vi "Main_TwoLoops.vi"() -> ()   [LabVIEW 2018]
uses:
  SubVIs/ENUMs/StateENUM.ctl
  <vilib>/Instr/_visa.llb/VISA Configure Serial Port (Instr).vi
  <vilib>/ptbypt/NI_PtbyPt.lvlib
panel:
  out "Waveform Chart":dbl(graph)
  in  "Check Center":bool
  out "Step":i32
  in  "Increase Step":bool
  in  "Decrease Step":bool
  out "Center":i32
  out "LoopCount":i32
  in  "Jitter Up":bool
  in  "Jitter Down":bool
  out "Command Buffer":string
  in  "stop":bool
  out "Current Time":timestamp format="%<%I:%M:%S %p | %m/%d/%y>T"
  in  "VISA resource name":refnum<visa-resource-name>="COM9"
  in  "Up Button":bool
  in  "Down Button":bool
  # "Manual\nAdjustment"
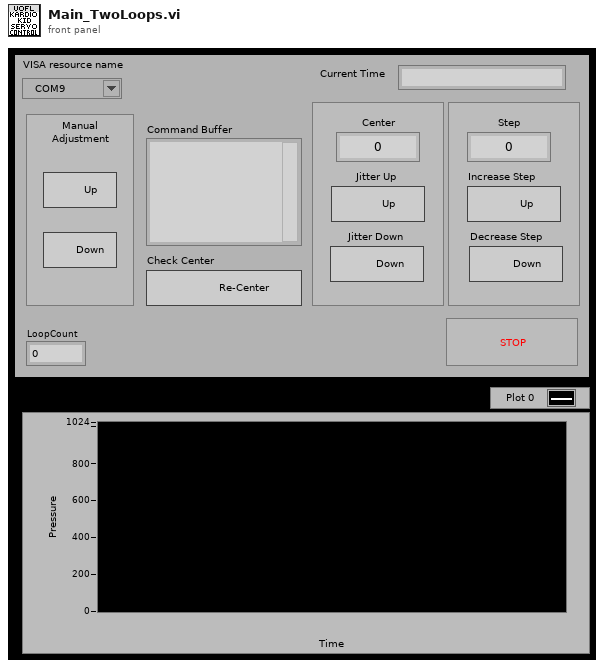
[diagram p1: front panel]
types:
  T1 = typedef "StateENUM.ctl" = enum16{"Init", "Idle", "MoveUp", "MoveDown", "JitterUp", "JitterDown", "IncreaseStep", "DecreaseStep", "CheckCenter", "ReadSerial", "ScanData", "Shutdown"}
  T2 = cluster{"State":T1, "Stop":bool, "error out":errorcluster}
  T3 = typedef "MoveCommands.ctl" = cluster{"MoveUp":string, "MoveDown":string, "JitterUp":string, "JitterDown":string, "IncStep":string, "DecStep":string, "ChkCenter":string}
  T4 = cluster{"VISA resource name out":refnum<visa-resource-name>, "error out":errorcluster, "State":T1, "Stop":bool, "Buffer":string, "Center":i32, "Step":i32, "SerialIncoming?":bool, "MoveCommands":T3}
  T5 = cluster{"Command Buffer":refnum<vi>, "Jitter Up":refnum<vi>, "Jitter Down":refnum<vi>, "Increase Step":refnum<vi>, "Decrease Step":refnum<vi>}
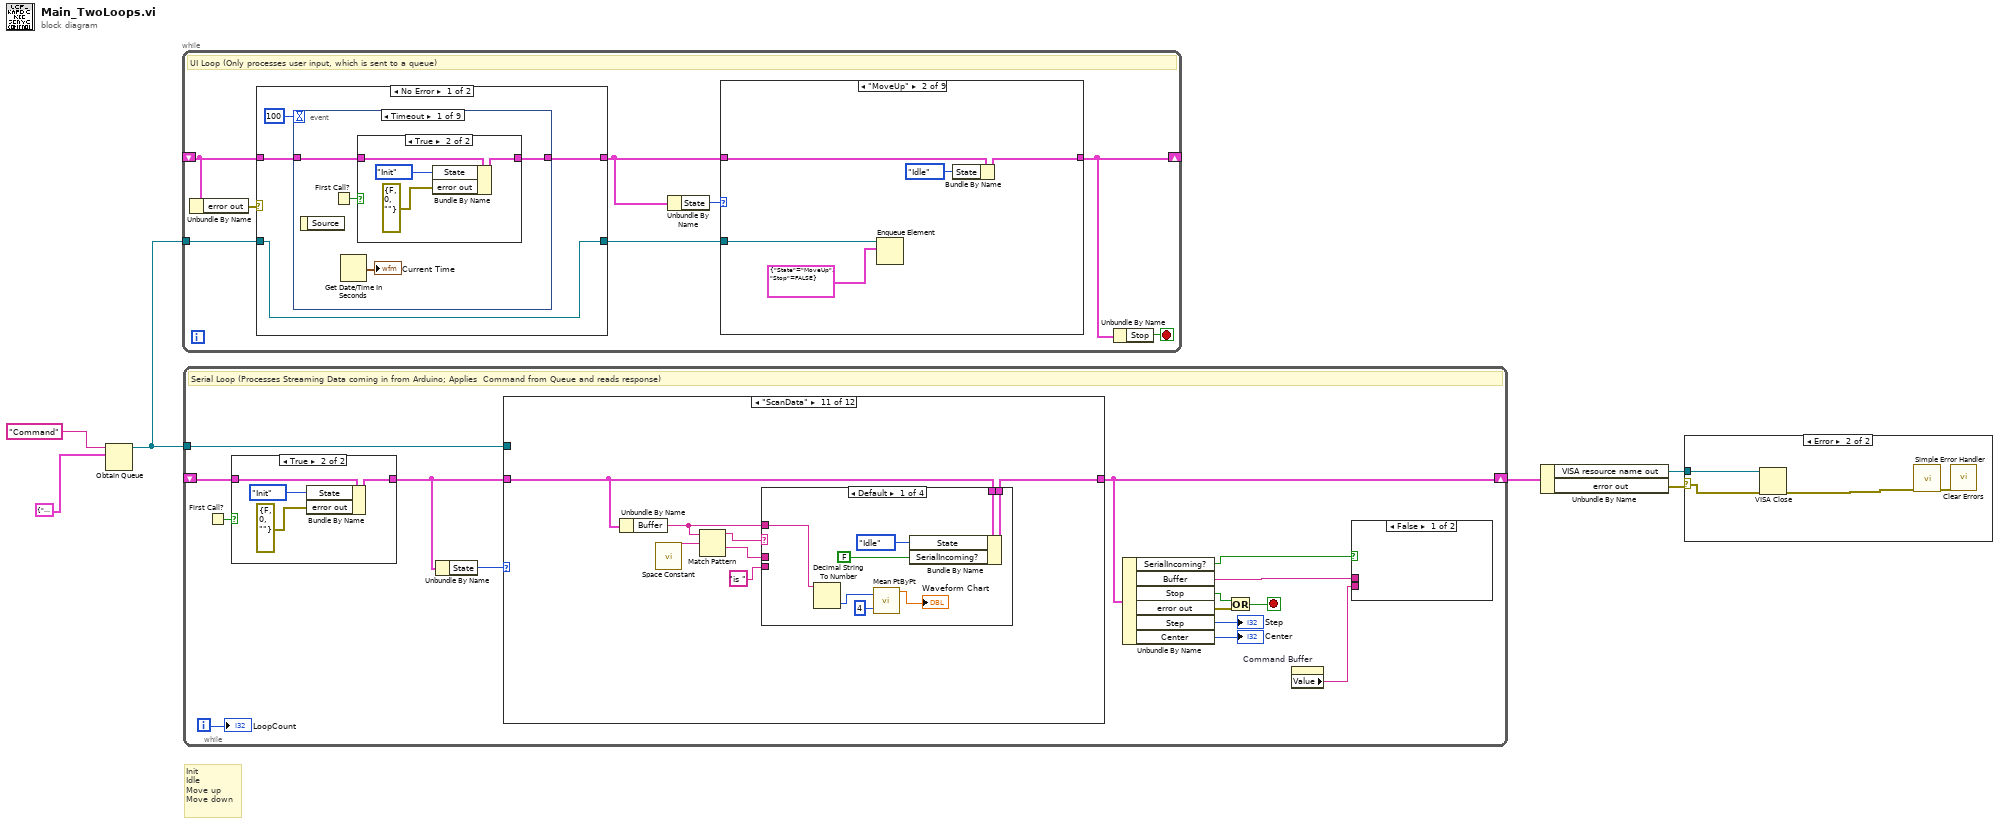
[diagram p0: block diagram]
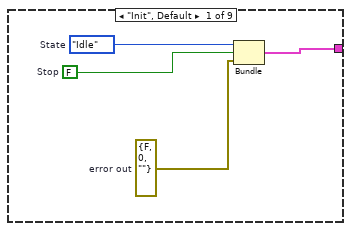
[diagram p2: hidden frame]
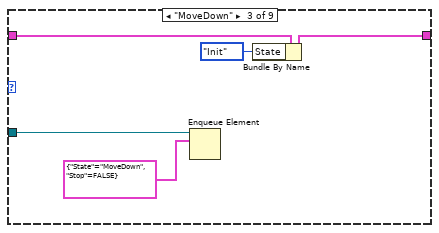
[diagram p3: hidden frame]
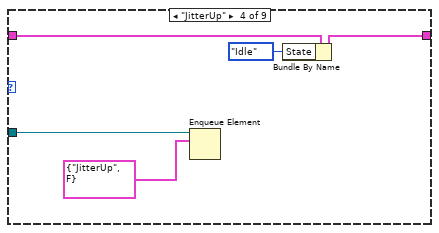
[diagram p4: hidden frame]
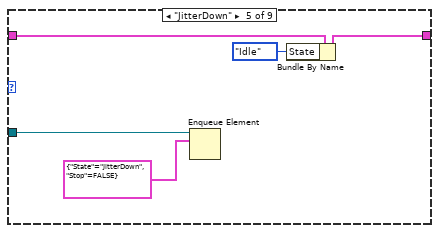
[diagram p5: hidden frame]
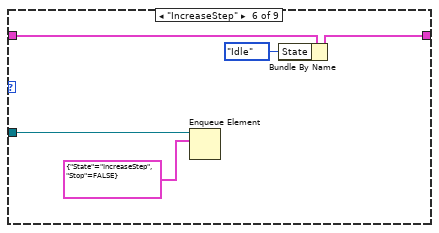
[diagram p6: hidden frame]
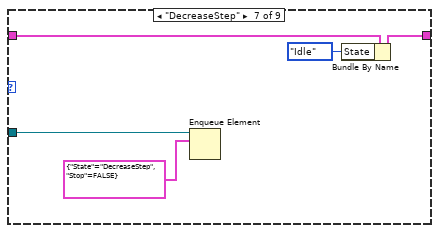
[diagram p7: hidden frame]
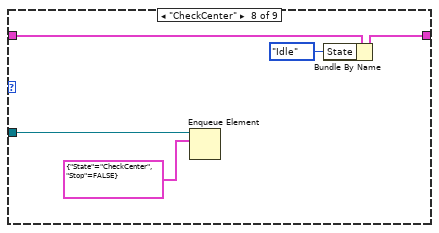
[diagram p8: hidden frame]
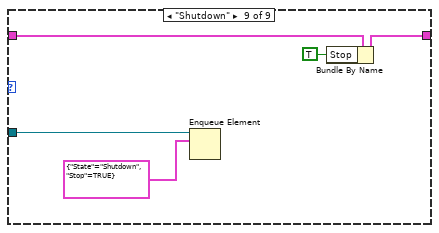
[diagram p9: hidden frame]
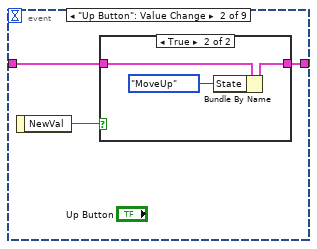
[diagram p11: hidden frame]
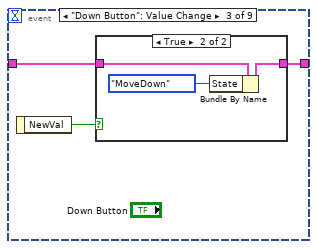
[diagram p13: hidden frame]
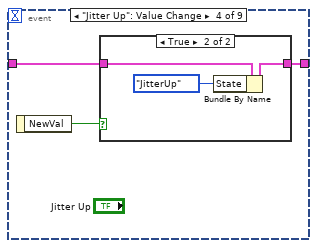
[diagram p15: hidden frame]
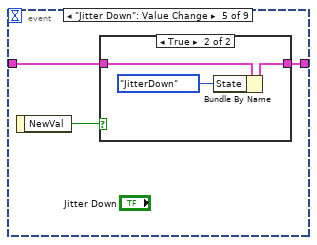
[diagram p17: hidden frame]
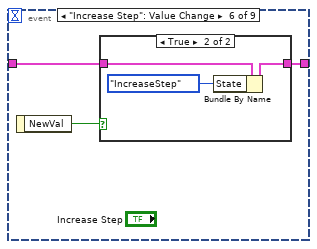
[diagram p19: hidden frame]
diagram:
  # "Init\nIdle\nMove up\nMove down"
  n1 = Obtain Queue(name (unnamed)="Command", element data type=cluster{"State":T1, "Stop":bool} {"State"=enum."ReadSerial", "Stop"=FALSE}) -> (queue out=w1:refnum<queue>)  [unwired: 3 in, 2 out]
  n2 = while {
    shift-right: [w13] -> _
    shift-left: _ -> [w10]
    tunnel: w1 -> [w8]
    stop <- w12 stop-if-true
    # "UI Loop (Only processes user input, which is sent to a queue)"
    n3 = Unbundle By Name(w10) -> ("error out"=w9:errorcluster)
    n4 = case shown="No Error" w9 {
      tunnel: w10 -> [w60 w134]
      tunnel: [w61 w130] -> w14
      tunnel: w8 -> [w59 w128]
      tunnel: [w59 w128] -> w7
      frame No Error {
        n5 = event shown="[0] Timeout" {
          selector: _ -> [_ _ _ _ _ _ _ _ _]
          dyn-events: _ -> [_ _ _ _ _ _ _ _ _]
          timeout: 100 -> [_ _ _ _ _ _ _ _ _]
          tunnel: w60 -> [w64 w74 w80 w88 w95 w102 w109 w116 w122]
          tunnel: [w63 w72 w79 w86 w93 w100 w107 w114 w121] -> w61
          event Timeout {
            n6 = event-data() -> ()  [unwired: 1 in, 1 out]
            n7 = First Call?() -> (First Call?: T/F=w65:bool)
            n8 = Get Date/Time In Seconds() -> (seconds since 1Jan1904=→"Current Time":timestamp)
            n9 = case shown="True" w65 {
              tunnel: [w67 w70] -> w63
              tunnel: w64 -> [w67 w71]
              frame False {
              }
              frame True {
                n10 = Bundle By Name(cluster=w71, "State"=StateENUM."Init", "error out"=errorcluster {"status"=FALSE, "code"=0, "source"=""}) -> (w70:T2)
              }
            }
          }
          event "Up Button": Value Change {
            n11 = event-data() -> ("NewVal"=w73:bool)  [unwired: 1 in]
            n12 = case shown="True" w73 {
              tunnel: w74 -> [w75 w78]
              tunnel: [w75 w77] -> w72
              frame False {
              }
              frame True {
                n13 = Bundle By Name(cluster=w78, "State"=StateENUM."MoveUp") -> (w77:T2)
              }
            }
          }
          event "Down Button": Value Change {
            n14 = event-data() -> ("NewVal"=w81:bool)  [unwired: 1 in]
            n15 = case shown="True" w81 {
              tunnel: w80 -> [w82 w85]
              tunnel: [w82 w84] -> w79
              frame False {
              }
              frame True {
                n16 = Bundle By Name(cluster=w85, "State"=StateENUM."MoveDown") -> (w84:T2)
              }
            }
          }
          event "Jitter Up": Value Change {
            n17 = event-data() -> ("NewVal"=w87:bool)  [unwired: 1 in]
            n18 = case shown="True" w87 {
              tunnel: w88 -> [w89 w92]
              tunnel: [w89 w91] -> w86
              frame False {
              }
              frame True {
                n19 = Bundle By Name(cluster=w92, "State"=StateENUM."JitterUp") -> (w91:T2)
              }
            }
          }
          event "Jitter Down": Value Change {
            n20 = event-data() -> ("NewVal"=w94:bool)  [unwired: 1 in]
            n21 = case shown="True" w94 {
              tunnel: w95 -> [w96 w99]
              tunnel: [w96 w98] -> w93
              frame False {
              }
              frame True {
                n22 = Bundle By Name(cluster=w99, "State"=StateENUM."JitterDown") -> (w98:T2)
              }
            }
          }
          event "Increase Step": Value Change {
            n23 = event-data() -> ("NewVal"=w101:bool)  [unwired: 1 in]
            n24 = case shown="True" w101 {
              tunnel: w102 -> [w103 w106]
              tunnel: [w103 w105] -> w100
              frame False {
              }
              frame True {
                n25 = Bundle By Name(cluster=w106, "State"=StateENUM."IncreaseStep") -> (w105:T2)
              }
            }
          }
          event "Decrease Step": Value Change {
            n26 = event-data() -> ("NewVal"=w108:bool)  [unwired: 1 in]
            n27 = case shown="True" w108 {
              tunnel: w109 -> [w110 w113]
              tunnel: [w110 w112] -> w107
              frame False {
              }
              frame True {
                n28 = Bundle By Name(cluster=w113, "State"=StateENUM."DecreaseStep") -> (w112:T2)
              }
            }
          }
          event "Check Center": Value Change {
            n29 = event-data() -> ("NewVal"=w115:bool)  [unwired: 1 in]
            n30 = case shown="True" w115 {
              tunnel: w116 -> [w117 w120]
              tunnel: [w117 w119] -> w114
              frame False {
              }
              frame True {
                n31 = Bundle By Name(cluster=w120, "State"=StateENUM."CheckCenter") -> (w119:T2)
              }
            }
          }
          event "stop": Value Change {
            n32 = event-data() -> ("NewVal"=w123:bool)  [unwired: 1 in]
            n33 = case shown="True" w123 {
              tunnel: w122 -> [w124 w127]
              tunnel: [w124 w126] -> w121
              frame False {
              }
              frame True {
                n34 = Bundle By Name(cluster=w127, "State"=StateENUM."Shutdown") -> (w126:T2)
              }
            }
          }
        }
      }
      frame Error {
        n35 = Unbundle By Name(w134) -> ("error out"=w133:errorcluster)
        n36 = call <vilib>:"Simple Error Handler.vi"("error in (no error)"=w133) -> ("code out"=w131:i32, "error out"=w132:errorcluster)  [unwired: 4 in, 3 out]
        n37 = call <vilib>:"Clear Errors.vi"("error in (no error)"=w132, "specific error code to clear (0: all)"=w131) -> ()  [unwired: 4 in, 2 out]
        n38 = Bundle By Name(cluster=w134, "State"=StateENUM."Shutdown") -> (w130:T2)
      }
    }
    n39 = Unbundle By Name(w14) -> ("State"=w11:T1)
    n40 = case shown="\"MoveUp\"" w11 {
      tunnel: w14 -> [_ w21 w26 w31 w36 w41 w46 w51 w56]
      tunnel: [w16 w20 w25 w30 w35 w40 w45 w50 w55] -> w13
      tunnel: w7 -> [_ w23 w28 w33 w38 w43 w48 w53 w58]
      frame "Init", Default {
        w15 = errorcluster {"status"=FALSE, "code"=0, "source"=""}  # error out
        w17 = FALSE  # Stop
        w18 = StateENUM."Idle"  # State
        n41 = Bundle("State"=w18, "Stop"=w17, "error out"=w15) -> (w16:T2)  [unwired: 1 in]
      }
      frame "MoveUp" {
        n42 = Enqueue Element(queue=w23, element=cluster{"State":T1, "Stop":bool} {"State"=enum."MoveUp", "Stop"=FALSE}) -> ()  [unwired: 2 in, 3 out]
        n43 = Bundle By Name(cluster=w21, "State"=StateENUM."Idle") -> (w20:T2)
      }
      frame "MoveDown" {
        n44 = Enqueue Element(queue=w28, element=cluster{"State":T1, "Stop":bool} {"State"=enum."MoveDown", "Stop"=FALSE}) -> ()  [unwired: 2 in, 3 out]
        n45 = Bundle By Name(cluster=w26, "State"=StateENUM."Init") -> (w25:T2)
      }
      frame "JitterUp" {
        n46 = Enqueue Element(queue=w33, element=cluster{"State":T1, "Stop":bool} {"State"=enum."JitterUp", "Stop"=FALSE}) -> ()  [unwired: 2 in, 3 out]
        n47 = Bundle By Name(cluster=w31, "State"=StateENUM."Idle") -> (w30:T2)
      }
      frame "JitterDown" {
        n48 = Enqueue Element(queue=w38, element=cluster{"State":T1, "Stop":bool} {"State"=enum."JitterDown", "Stop"=FALSE}) -> ()  [unwired: 2 in, 3 out]
        n49 = Bundle By Name(cluster=w36, "State"=StateENUM."Idle") -> (w35:T2)
      }
      frame "IncreaseStep" {
        n50 = Enqueue Element(queue=w43, element=cluster{"State":T1, "Stop":bool} {"State"=enum."IncreaseStep", "Stop"=FALSE}) -> ()  [unwired: 2 in, 3 out]
        n51 = Bundle By Name(cluster=w41, "State"=StateENUM."Idle") -> (w40:T2)
      }
      frame "DecreaseStep" {
        n52 = Enqueue Element(queue=w48, element=cluster{"State":T1, "Stop":bool} {"State"=enum."DecreaseStep", "Stop"=FALSE}) -> ()  [unwired: 2 in, 3 out]
        n53 = Bundle By Name(cluster=w46, "State"=StateENUM."Idle") -> (w45:T2)
      }
      frame "CheckCenter" {
        n54 = Enqueue Element(queue=w53, element=cluster{"State":T1, "Stop":bool} {"State"=enum."CheckCenter", "Stop"=FALSE}) -> ()  [unwired: 2 in, 3 out]
        n55 = Bundle By Name(cluster=w51, "State"=StateENUM."Idle") -> (w50:T2)
      }
      frame "Shutdown" {
        n56 = Enqueue Element(queue=w58, element=cluster{"State":T1, "Stop":bool} {"State"=enum."Shutdown", "Stop"=TRUE}) -> ()  [unwired: 2 in, 3 out]
        n57 = Bundle By Name(cluster=w56, "Stop"=TRUE) -> (w55:T2)
      }
    }
    n58 = Unbundle By Name(w13) -> ("Stop"=w12:bool)
  }
  n59 = while {
    shift-right: [w148] -> w6
    shift-left: _ -> [w137]
    tunnel: w1 -> [w135]
    i -> [w147]
    stop <- w146 stop-if-true
    # "Serial Loop (Processes Streaming Data coming in from Arduino; Applies  Command from Queue and reads response)"
    n60 = First Call?() -> (First Call?: T/F=w138:bool)
    n61 = case shown="True" w138 {
      tunnel: [w150 w153] -> w136
      tunnel: w137 -> [w150 w154]
      frame False {
      }
      frame True {
        n62 = Bundle By Name(cluster=w154, "State"=StateENUM."Init", "error out"=errorcluster {"status"=FALSE, "code"=0, "source"=""}) -> (w153:T4)
      }
    }
    n63 = Unbundle By Name(w136) -> ("State"=w149:T1)
    n64 = case shown="\"ScanData\"" w149 {
      tunnel: [w178 w183 w206 w213 w221 w230 w237 w244 w251 w266 w284 w323] -> w148
      tunnel: w136 -> [_ w184 w207 w214 w223 w232 w239 w246 w253 w267 w285 w325]
      tunnel: w135 -> [_ w182 _ _ _ _ _ _ _ _ _ w318]
      frame "Init", Default {
        w166 = FALSE  # SerialIncoming?
        w168 = 50  # Step
        w169 = 1500  # Center
        w171 = ""  # Buffer
        w176 = FALSE  # Stop
        w177 = StateENUM."Idle"  # State
        n65 = property on="Command Buffer" class="Str"("Value"="") -> ()  [unwired: 2 in, 2 out]
        n66 = call-poly "VISA Configure Serial Port"("VISA resource name"="VISA resource name") -> ("VISA resource name out"=w174:refnum<visa-resource-name>, "error out"=w173:errorcluster)  [unwired: 13 in]
        n67 = VISA Flush I/O Buffer(VISA resource name=w174, error in (no error)=w173) -> (VISA resource name out=w167:refnum<visa-resource-name>, error out=w172:errorcluster)  [unwired: 1 in]
        n68 = control-ref of="Jitter Up"() -> (w161:refnum<vi>)
        n69 = control-ref of="Jitter Down"() -> (w162:refnum<vi>)
        n70 = control-ref of="Increase Step"() -> (w163:refnum<vi>)
        n71 = control-ref of="Decrease Step"() -> (w164:refnum<vi>)
        n72 = control-ref of="Command Buffer"() -> (w160:refnum<vi>)
        n73 = Bundle("Command Buffer"=w160, "Jitter Up"=w161, "Jitter Down"=w162, "Increase Step"=w163, "Decrease Step"=w164) -> (w159:T5)  [unwired: 1 in]
        n74 = call "MoveCommands (SubVI).vi"() -> ("MoveCommands"=w165:T3)  [unwired: 11 in]
        n75 = call "InitPostions (SubVI).vi"("ControlCluster"=w159) -> ()  [unwired: 11 in]
        n76 = Wait (ms)(milliseconds to wait=u32 5) -> ()  [unwired: 1 out]
        n77 = Bundle("VISA resource name out"=w167, "error out"=w172, "State"=w177, "Stop"=w176, "Buffer"=w171, "Center"=w169, "Step"=w168, "SerialIncoming?"=w166, "MoveCommands"=w165) -> (w178:T4)  [unwired: 1 in]
      }
      frame "Idle" {
        n78 = Dequeue Element(queue=w182, timeout in ms (-1)=10) -> (element=w180:cluster{"State":T1, "Stop":bool}, timed out?=w181:bool)  [unwired: 1 in, 2 out]
        n79 = case shown="False" w181 {
          tunnel: w184 -> [w188 w200]
          tunnel: [w187 w198] -> w183
          tunnel: w180 -> [w186 _]
          frame False {
            n80 = Unbundle By Name(w186) -> ("State"=w185:T1)
            n81 = Bundle By Name(cluster=w188, "State"=w185) -> (w187:T4)
          }
          frame True {
            w192 = StateENUM."ReadSerial"  # State
            n82 = Unbundle By Name(w200) -> ("State"=w191:T1, "VISA resource name out"=w197:refnum<visa-resource-name>, "error out"=w196:errorcluster)
            n83 = Wait (ms)(milliseconds to wait=u32 5) -> ()  [unwired: 1 out]
            n84 = property class="Instr"(reference=w197, error in=w196) -> (error out=w195:errorcluster, "Serial Settings:Number of Bytes at Serial Port"=w193:u32)  [unwired: 1 out]
            n85 = Greater Than 0?(x=w193) -> (x > 0?=w190:bool)
            n86 = Select(t=w192, s=w190, f=w191) -> (s? t:f=w194:T1)
            n87 = Bundle By Name(cluster=w200, "State"=w194, "error out"=w195, "SerialIncoming?"=FALSE) -> (w198:T4)
          }
        }
      }
      frame "MoveUp" {
        # "48 ASCII"
        n88 = Unbundle By Name(w207) -> ("VISA resource name out"=w202:refnum<visa-resource-name>, "MoveCommands.MoveUp"=w201:string, "error out"=w203:errorcluster)
        n89 = VISA Write(VISA resource name=w202, write buffer=w201, error in (no error)=w203) -> (error out=w204:errorcluster)  [unwired: 2 out]
        n90 = Bundle By Name(cluster=w207, "State"=StateENUM."ReadSerial", "error out"=w204) -> (w206:T4)
      }
      frame "MoveDown" {
        # "49 ASCII"
        n91 = Unbundle By Name(w214) -> ("VISA resource name out"=w209:refnum<visa-resource-name>, "MoveCommands.MoveDown"=w208:string, "error out"=w210:errorcluster)
        n92 = VISA Write(VISA resource name=w209, write buffer=w208, error in (no error)=w210) -> (error out=w211:errorcluster)  [unwired: 2 out]
        n93 = Bundle By Name(cluster=w214, "State"=StateENUM."ReadSerial", "error out"=w211) -> (w213:T4)
      }
      frame "JitterUp" {
        n94 = Unbundle By Name(w223) -> ("Center"=w218:i32, "VISA resource name out"=w222:refnum<visa-resource-name>, "MoveCommands.JitterUp"=w215:string, "error out"=w216:errorcluster)
        n95 = Increment(x=w218) -> (x+1=w217:i32)
        n96 = VISA Write(VISA resource name=w222, write buffer=w215, error in (no error)=w216) -> (error out=w219:errorcluster)  [unwired: 2 out]
        n97 = Bundle By Name(cluster=w223, "State"=StateENUM."ReadSerial", "Center"=w217, "error out"=w219) -> (w221:T4)
      }
      frame "JitterDown" {
        n98 = Unbundle By Name(w232) -> ("Center"=w227:i32, "VISA resource name out"=w231:refnum<visa-resource-name>, "MoveCommands.JitterDown"=w224:string, "error out"=w225:errorcluster)
        n99 = Decrement(x=w227) -> (x-1=w226:i32)
        n100 = VISA Write(VISA resource name=w231, write buffer=w224, error in (no error)=w225) -> (error out=w228:errorcluster)  [unwired: 2 out]
        n101 = Bundle By Name(cluster=w232, "State"=StateENUM."ReadSerial", "Center"=w226, "error out"=w228) -> (w230:T4)
      }
      frame "IncreaseStep" {
        n102 = Unbundle By Name(w239) -> ("VISA resource name out"=w238:refnum<visa-resource-name>, "MoveCommands.IncStep"=w233:string, "error out"=w234:errorcluster)
        n103 = VISA Write(VISA resource name=w238, write buffer=w233, error in (no error)=w234) -> (error out=w235:errorcluster)  [unwired: 2 out]
        n104 = Bundle By Name(cluster=w239, "State"=StateENUM."ReadSerial", "error out"=w235) -> (w237:T4)
      }
      frame "DecreaseStep" {
        n105 = Unbundle By Name(w246) -> ("VISA resource name out"=w245:refnum<visa-resource-name>, "MoveCommands.DecStep"=w241:string, "error out"=w240:errorcluster)
        n106 = VISA Write(VISA resource name=w245, write buffer=w241, error in (no error)=w240) -> (error out=w242:errorcluster)  [unwired: 2 out]
        n107 = Bundle By Name(cluster=w246, "State"=StateENUM."ReadSerial", "error out"=w242) -> (w244:T4)
      }
      frame "CheckCenter" {
        n108 = Unbundle By Name(w253) -> ("VISA resource name out"=w252:refnum<visa-resource-name>, "MoveCommands.ChkCenter"=w247:string, "error out"=w248:errorcluster)
        n109 = VISA Write(VISA resource name=w252, write buffer=w247, error in (no error)=w248) -> (error out=w249:errorcluster)  [unwired: 2 out]
        n110 = Bundle By Name(cluster=w253, "State"=StateENUM."ReadSerial", "error out"=w249) -> (w251:T4)
      }
      frame "ReadSerial" {
        n111 = Unbundle By Name(w267) -> ("VISA resource name out"=w262:refnum<visa-resource-name>, "error out"=w257:errorcluster, "Buffer"=w256:string)
        n112 = Wait (ms)(milliseconds to wait=u32 5) -> ()  [unwired: 1 out]
        n113 = property class="Instr"(reference=w262, error in=w257) -> (reference out=w259:refnum<visa-resource-name>, error out=w258:errorcluster, "Serial Settings:Number of Bytes at Serial Port"=w260:u32)
        n114 = Greater Than 0?(x=w260) -> (x > 0?=w261:bool)
        n115 = case shown="True" w261 {
          tunnel: [w270 w278] -> w264
          tunnel: [w271 w277] -> w263
          tunnel: w258 -> [w271 w276]
          tunnel: w259 -> [_ w275]
          tunnel: w260 -> [_ w274]
          tunnel: w256 -> [w270 _]
          tunnel: [StateENUM."Idle" ("State") StateENUM."ScanData" ("State")] -> w255
          tunnel: [FALSE FALSE] -> w254
          frame False {
          }
          frame True {
            n116 = VISA Read(VISA resource name=w275, byte count=w274, error in (no error)=w276) -> (read buffer=w278:string, error out=w277:errorcluster)  [unwired: 2 out]
          }
        }
        n117 = Bundle By Name(cluster=w267, "State"=w255, "SerialIncoming?"=w254, "Buffer"=w264, "error out"=w263) -> (w266:T4)
      }
      frame "ScanData" {
        n118 = Unbundle By Name(w285) -> ("Buffer"=w279:string)
        n119 = call <vilib>:"Space Constant.vi"() -> ("String"=w281:string)
        n120 = Match Pattern(string=w279, regular expression=w281) -> (before substring=w280:string, after substring=w282:string)  [unwired: 1 in, 2 out]
        n121 = case shown="Default" w280 {
          tunnel: "is " -> [_ _ w307 w317]
          tunnel: w282 -> [_ _ w306 w316]
          tunnel: w285 -> [w293 w297 w302 w312]
          tunnel: [w292 w296 w300 w310] -> w284
          tunnel: w279 -> [w289 _ _ _]
          frame Default {
            n122 = Decimal String To Number(string=w289) -> (number=w287:i32)  [unwired: 2 in, 1 out]
            n123 = call <vilib>:"Mean PtByPt.vi"("x"=w287, "sample length"=4) -> ("mean"=→"Waveform Chart":dbl)  [unwired: 2 in, 1 out]
            n124 = Bundle By Name(cluster=w293, "State"=StateENUM."Idle", "SerialIncoming?"=FALSE) -> (w292:T4)
          }
          frame "Moving" {
            n125 = Bundle By Name(cluster=w297, "State"=StateENUM."Idle", "SerialIncoming?"=TRUE) -> (w296:T4)
          }
          frame "Center", "Stop" {
            n126 = Match Pattern(string=w306, regular expression=w307) -> (after substring=w304:string)  [unwired: 1 in, 3 out]
            n127 = Match Pattern(string=w304, regular expression="\r\n") -> (before substring=w303:string)  [unwired: 1 in, 3 out]
            n128 = Decimal String To Number(string=w303) -> (number=w301:i32)  [unwired: 2 in, 1 out]
            n129 = Bundle By Name(cluster=w302, "SerialIncoming?"=TRUE, "State"=StateENUM."Idle", "Center"=w301) -> (w300:T4)
          }
          frame "Step" {
            n130 = Match Pattern(string=w316, regular expression=w317) -> (after substring=w314:string)  [unwired: 1 in, 3 out]
            n131 = Match Pattern(string=w314, regular expression="\r\n") -> (before substring=w313:string)  [unwired: 1 in, 3 out]
            n132 = Decimal String To Number(string=w313) -> (number=w311:i32)  [unwired: 2 in, 1 out]
            n133 = Bundle By Name(cluster=w312, "SerialIncoming?"=TRUE, "State"=StateENUM."Idle", "Step"=w311) -> (w310:T4)
          }
        }
      }
      frame "Shutdown" {
        n134 = Release Queue(queue=w318) -> ()  [unwired: 2 in, 3 out]
        n135 = Unbundle By Name(w325) -> ("VISA resource name out"=w324:refnum<visa-resource-name>, "error out"=w319:errorcluster)
        n136 = VISA Close(VISA resource name=w324, error in (no error)=w319) -> (error out=w320:errorcluster)
        n137 = Bundle By Name(cluster=w325, "Stop"=TRUE, "State"=StateENUM."Shutdown", "error out"=w320) -> (w323:T4)
      }
    }
    n138 = Unbundle By Name(w148) -> ("SerialIncoming?"=w139:bool, "Buffer"=w143:string, "Stop"=w145:bool, "error out"=w144:errorcluster, "Step"=→"Step":i32, "Center"=→"Center":i32)
    n139 = Or(x=w145, y=w144) -> (x .or. y?=w146:bool)
    n140 = property on="Command Buffer" class="Str"() -> ("Value"=w142:string)  [unwired: 2 in, 2 out]
    n141 = case shown="False" w139 {
      tunnel: w143 -> [_ w157]
      tunnel: w142 -> [_ w156]
      frame False {
      }
      frame True {
        n142 = Concatenate Strings(w157, w156) -> (→"Command Buffer":string)
      }
    }
    "LoopCount" <- w147
  }
  n143 = Unbundle By Name(w6) -> ("VISA resource name out"=w4:refnum<visa-resource-name>, "error out"=w5:errorcluster)
  n144 = case shown="Error" w5 {
    selector: w5 -> [_ w327]
    tunnel: w4 -> [_ w329]
    frame No Error {
    }
    frame Error {
      n145 = VISA Close(VISA resource name=w329, error in (no error)=w327) -> (error out=w326:errorcluster)
      n146 = call <vilib>:"Simple Error Handler.vi"("error in (no error)"=w326) -> ("error out"=w328:errorcluster)  [unwired: 4 in, 4 out]
      n147 = call <vilib>:"Clear Errors.vi"("error in (no error)"=w328) -> ()  [unwired: 5 in, 2 out]
    }
  }
